vi "Flush Port.vi"(8 "error in (no error)":errorcluster, 10 "Port":T1="Mod6\\Port1", 11 "TestMPU in":refnum<class "TestMPU.lvclass">) -> (0 "error out":errorcluster, 3 "TestMPU out":refnum<class "TestMPU.lvclass">)   [LabVIEW 2018, in "TestMPU.lvclass"]
uses:
  TestMPU.lvclass
  src/PortType.ctl
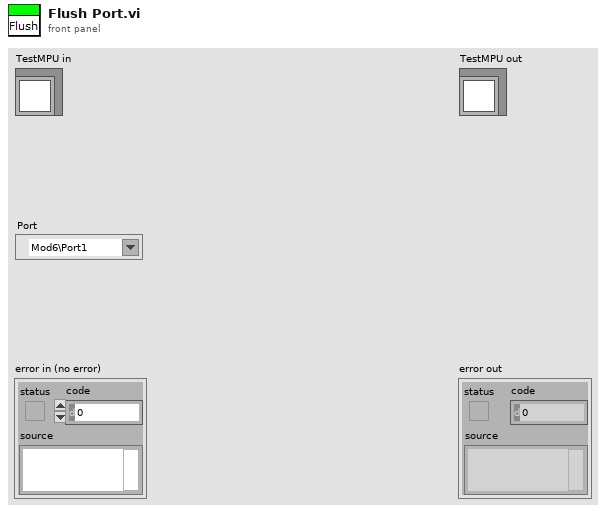
[diagram p1: front panel]
types:
  T1 = typedef "PortType.ctl" = refnum<k21>
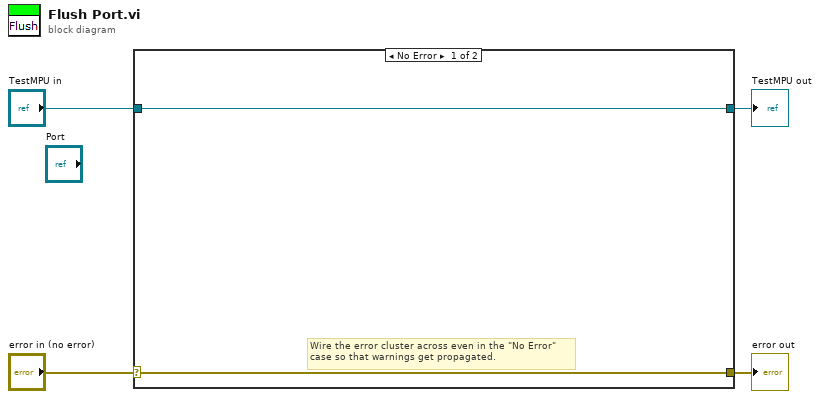
[diagram p0: block diagram]
diagram:
  n1 = case shown="No Error" "error in (no error)" {
    selector: "error in (no error)" -> [w5 w8]
    tunnel: [w5 w8] -> w3
    tunnel: [w6 w7] -> w1
    tunnel: "TestMPU in" -> [w6 w7]
    frame No Error {
      # "Wire the error cluster across even in the \"No Error\"\ncase so that warnings get propagated."
    }
    frame Error {
    }
  }
  "error out" <- w3
  "TestMPU out" <- w1
